vi "Fault_ID_Parse_FL24_Dryer.vi"(8 "Enum":enum16{"Sequence", "Table"}(ring), 11 "Numeric":u32) -> (3 "String":string)   [LabVIEW 2016]
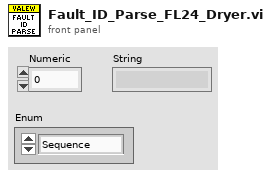
[diagram p1: front panel]
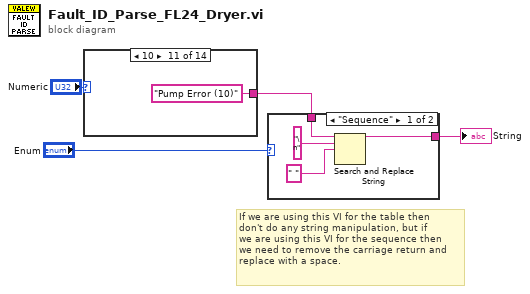
[diagram p0: block diagram]
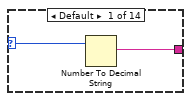
[diagram p3: hidden frame]
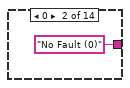
[diagram p4: hidden frame]
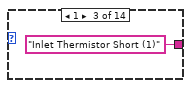
[diagram p5: hidden frame]
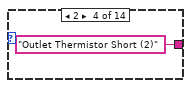
[diagram p6: hidden frame]
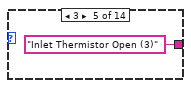
[diagram p7: hidden frame]
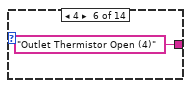
[diagram p8: hidden frame]
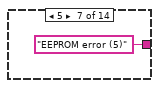
[diagram p9: hidden frame]
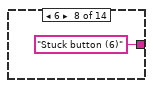
[diagram p10: hidden frame]
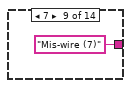
[diagram p11: hidden frame]
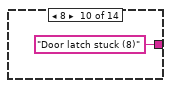
[diagram p12: hidden frame]
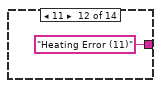
[diagram p13: hidden frame]
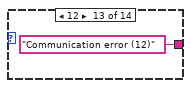
[diagram p14: hidden frame]
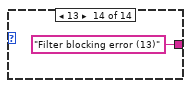
[diagram p15: hidden frame]
diagram:
  # "If we are using this VI for the table then\ndon't do any string manipulation, but if\nwe are using this VI for the sequence then\nwe need to remove the carriage return and\nreplace with a space."
  n1 = case shown="10" "Numeric" {
    selector: "Numeric" -> [w6 _ _ _ _ _ _ _ _ _ _ _ _ _]
    tunnel: [w5 "No Fault (0)" "Inlet Thermistor Short (1)" "Outlet Thermistor Short (2)" "Inlet Thermistor Open (3)" "Outlet Thermistor Open (4)" "EEPROM error (5)" "Stuck button (6)" "Mis-wire (7)" "Door latch stuck (8)" "Pump Error (10)" "Heating Error (11)" "Communication error (12)" "Filter blocking error (13)"] -> w3
    frame Default {
      n2 = Number To Decimal String(number=w6) -> (decimal integer string=w5:string)  [unwired: 1 in]
    }
    frame 0 {
    }
    frame 1 {
    }
    frame 2 {
    }
    frame 3 {
    }
    frame 4 {
    }
    frame 5 {
    }
    frame 6 {
    }
    frame 7 {
    }
    frame 8 {
    }
    frame 10 {
    }
    frame 11 {
    }
    frame 12 {
    }
    frame 13 {
    }
  }
  n3 = case shown="\"Sequence\"" "Enum" {
    tunnel: w3 -> [w23 w24]
    tunnel: [w20 w24] -> w2
    frame "Sequence" {
      n4 = Search and Replace String(input string=w23, search string="\n", replace string=" " ("replace string (\"\")")) -> (result string=w20:string)  [unwired: 5 in, 3 out]
    }
    frame "Table" {
    }
  }
  "String" <- w2
